vi "Open Hardware.vi"(8 "error in (no error)":errorcluster, 11 "Inst.TSL210 in":refnum<class "Inst.TSL210.lvclass">) -> (0 "error out":errorcluster, 3 "Inst.TSL210 out":refnum<class "Inst.TSL210.lvclass">)   [LabVIEW 2019, in "Inst.TSL210.lvclass"]
uses:
  Inst.TSL210.lvclass
  Inst.TSL210.lvclass/Inst.TSL210.ctl
  <userlib>/LevyLab/Instrument Framework/Instrument Types/VSource/Instrument.VSource.lvclass
  <userlib>/LevyLab/Instrument Framework/SMOs/Instrument/Instrument.lvclass
  C:/Program Files (x86)/National Instruments/LabVIEW 2019/user.lib/LevyLab/Instrument Framework/SMOs/Instrument/Instrument.lvclass
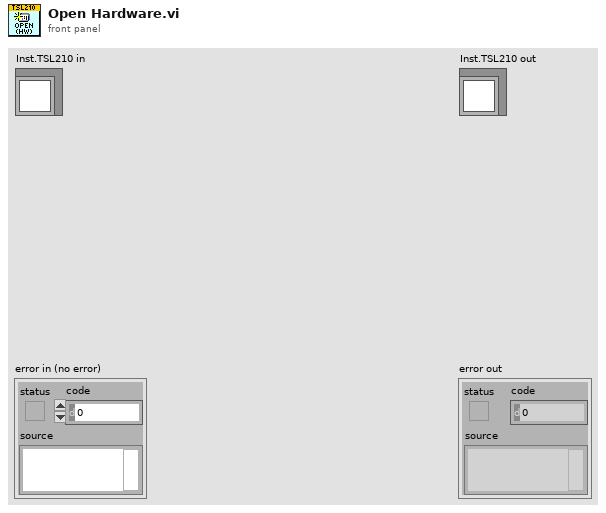
[diagram p1: front panel]
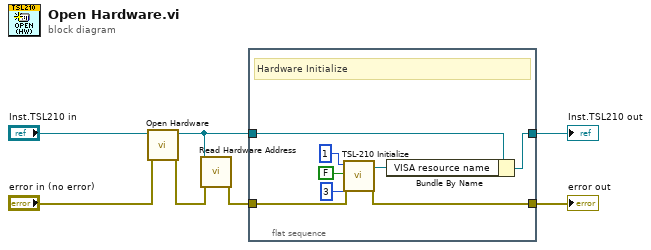
[diagram p0: block diagram]
diagram:
  n1 = call-parent "Open Hardware.vi"("error in (no error)"="error in (no error)", "Instrument in"="Inst.TSL210 in") -> ("error out"=w5:errorcluster, "Instrument out"=w4:refnum<class "Inst.TSL210.lvclass">)  [unwired: 8 in]
  n2 = call <userlib>:"Read Hardware Address.vi"("error in (no error)"=w5, "Instrument in"=w4) -> ("error out"=w2:errorcluster)  [unwired: 7 in, 2 out]
  n3 = flat-sequence {
    tunnel: w4 -> [w15]
    tunnel: [w8] -> w3
    tunnel: w2 -> [w12]
    tunnel: [w13] -> w1
    frame #0 {
      # "Hardware Initialize"
      n4 = call "TSL-210 Initialize.vi"("error in (no error)"=w12, "Termination Charactor"=3, "Reset (T: yes)"=FALSE, "GPIB address default: 5"=i16 1) -> ("error out"=w13:errorcluster, "dup VISA session"=w14:refnum<visa-resource-name>)  [unwired: 1 out]
      n5 = Bundle By Name(cluster=w15, "VISA resource name"=w14) -> (w8:refnum<class "Inst.TSL210.lvclass">)
    }
  }
  "error out" <- w1
  "Inst.TSL210 out" <- w3
